vi "DataLog_Update.vi"() -> ()   [LabVIEW 2018]
panel:
  out "레코드":T1(array[cluster])
  in  "version 폴더 경로":path
  in  "정지 버튼":bool
  in  "업로드버튼":bool
  in  "업로드할 파일 정보 입력란":T2
  in  "데이터로그 경로(대화 상자 사용)":path
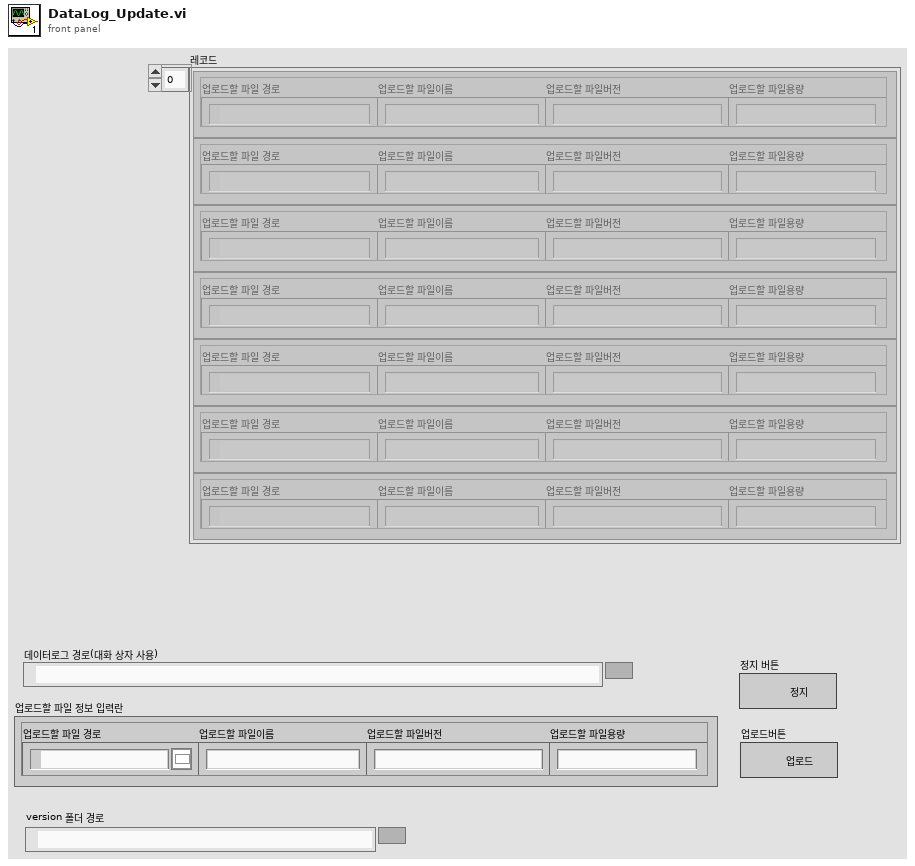
[diagram p1: front panel]
types:
  T1 = cluster{"업로드할 파일 경로":path, "업로드할 파일이름":string, "업로드할 파일버전":string, "업로드할 파일용량":string}[]
  T2 = cluster{"업로드할 파일 경로":path, "업로드할 파일이름":string, "업로드할 파일버전":string, "업로드할 파일용량":string}
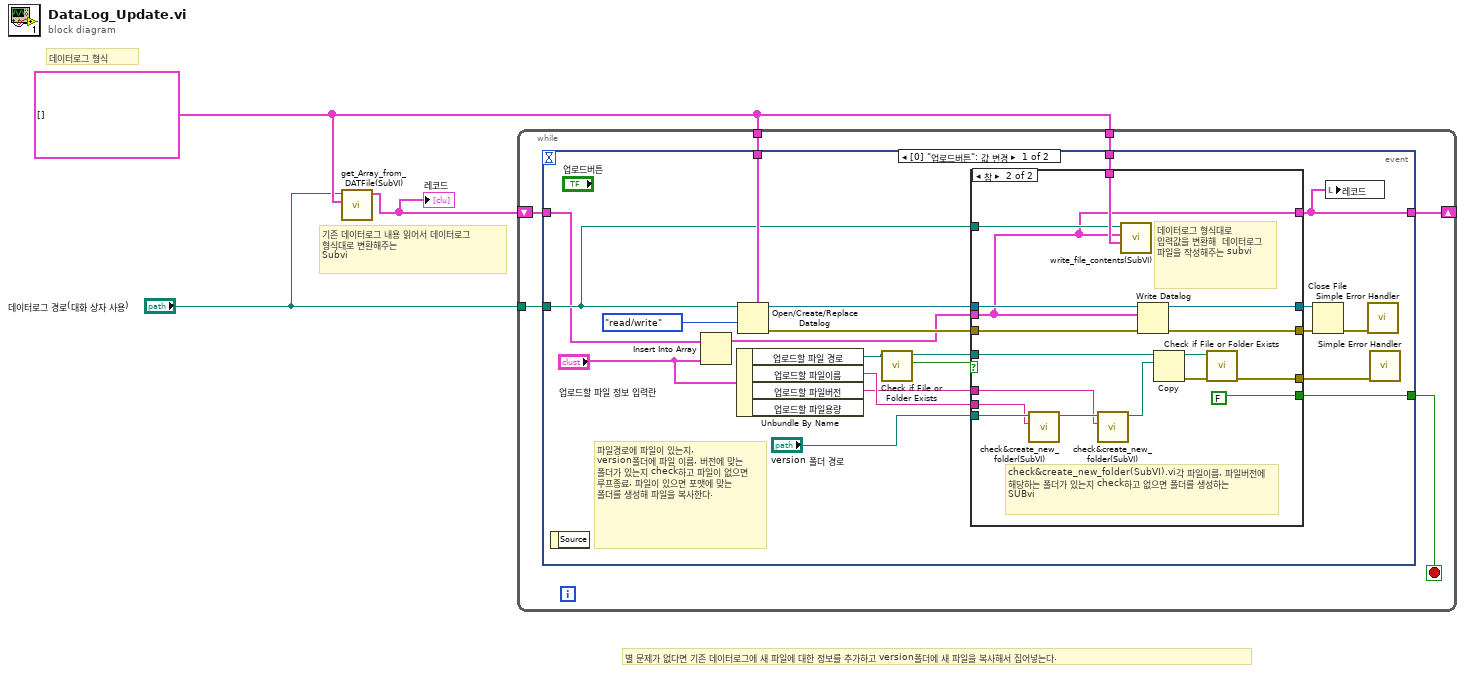
[diagram p0: block diagram]
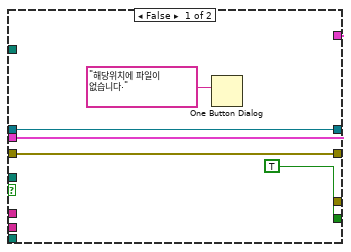
[diagram p2: hidden frame]
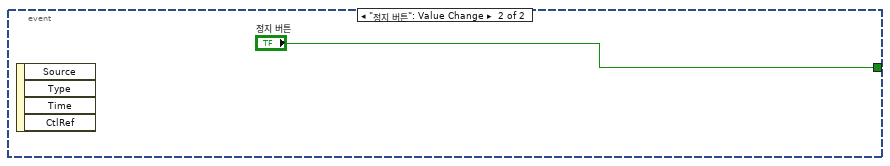
[diagram p3: hidden frame]
diagram:
  w3 = T1 [] ("레코드 2")
  # "데이터로그 형식"
  # "기존 데이터로그 내용 읽어서 데이터로그 형식대로 변환해주는\nSubvi"
  # "별 문제가 없다면 기존 데이터로그에 새 파일에 대한 정보를 추가하고 version폴더에 새 파일을 복사해서 집어넣는다."
  n1 = call "get_Array_from_DATFile(SubVI).vi"("레코드 3"=w3, "데이터로그 경로(대화 상자 사용)"="데이터로그 경로(대화 상자 사용)") -> ("레코드 2"=w1:T1)  [unwired: 9 in]
  "레코드" <- w1
  n2 = while {
    tunnel: w3 -> [w8]
    tunnel: "데이터로그 경로(대화 상자 사용)" -> [w7]
    tunnel: w3 -> [w6]
    shift-right: [w5] -> _
    shift-left: w1 -> [w4]
    stop <- w9 stop-if-true
    n3 = event shown="[0] \"업로드버튼\": 값 변경" {
      selector: _ -> [_ _]
      dyn-events: _ -> [_ _]
      timeout: _ -> [_ _]
      tunnel: [w19 "정지 버튼"] -> w9
      tunnel: w8 -> [w30 _]
      tunnel: w7 -> [w12 _]
      tunnel: w6 -> [w16 _]
      tunnel: w4 -> [w10 _]
      tunnel: [w11 _] -> w5
      event "업로드버튼": Value Change {
        # "파일경로에 파일이 있는지, \nversion폴더에 파일 이름, 버전에 맞는 폴더가 있는지 check하고 파일이 없으면 루프종료, 파일이 있으면 포맷에 맞는 폴더를 생성해 파일을 복사한다."
        n4 = event-data() -> ()  [unwired: 1 in, 1 out]
        n5 = Insert Into Array(array=w10, new element="업로드할 파일 정보 입력란") -> (w17:T1)  [unwired: 1 in]
        n6 = Unbundle By Name("업로드할 파일 정보 입력란") -> ("업로드할 파일 경로"=w13:path, "업로드할 파일이름"=w27:string, "업로드할 파일버전"=w26:string)  [unwired: 1 out]
        n7 = Open/Create/Replace Datalog(5:w30, 9:enum16{"read/write", "read-only", "write-only"}."read/write" ("접근(0:read/write)"), 11:w12) -> (0:w25:errorcluster, 3:w24:refnum<k1>)  [unwired: 3 in, 1 out]
        n8 = call <vilib>:"Check if File or Folder Exists.vi"("path"=w13) -> ("file or folder exists?"=w15:bool, "dup path"=w21:path)  [unwired: 8 in, 1 out]
        n9 = case shown="참" w15 {
          tunnel: [TRUE FALSE] -> w19
          tunnel: "version 폴더 경로" -> [_ w51]
          tunnel: w27 -> [_ w38]
          tunnel: w26 -> [_ w39]
          tunnel: w25 -> [w34 w49]
          tunnel: w17 -> [w31 w36]
          tunnel: w24 -> [w35 w48]
          tunnel: [w34 w47] -> w23
          tunnel: [w35 w46] -> w22
          tunnel: w21 -> [_ w44]
          tunnel: [_ w41] -> w20
          tunnel: w16 -> [_ w40]
          tunnel: w12 -> [_ w37]
          tunnel: [w31 w36] -> w11
          frame False {
            n10 = One Button Dialog(message="해당위치에 파일이 없습니다." ("메시지")) -> ()  [unwired: 1 in, 1 out]
          }
          frame True {
            # "데이터로그 형식대로 입력값을 변환해  데이터로그 파일을 작성해주는 subvi"
            # "check&create_new_folder(SubVI).vi각 파일이름, 파일버전에 해당하는 폴더가 있는지 check하고 없으면 폴더를 생성하는 SUBvi"
            n11 = call "check&create_new_folder(SubVI).vi"("업로드할 파일이름"=w38, "version 폴더 경로"=w51) -> ("dup path"=w50:path)  [unwired: 9 in]
            n12 = call "check&create_new_folder(SubVI).vi"("업로드할 파일이름"=w39, "version 폴더 경로"=w50) -> ("dup path"=w45:path)  [unwired: 9 in]
            n13 = call "write_file_contents(SubVI).vi"("레코드 3"=w40, "레코드 입력"=w36, "데이터로그 경로(대화 상자 사용)"=w37) -> ()  [unwired: 9 in]
            n14 = Write Datalog(4:w49, 6:w36, 7:w48) -> (0:w47:errorcluster, 3:w46:refnum<k1>)
            n15 = Copy(10:w45, 11:w44) -> (0:w42:errorcluster, 3:w43:path)  [unwired: 3 in, 1 out]
            n16 = call <vilib>:"Check if File or Folder Exists.vi"("error in (no error)"=w42, "path"=w43) -> ("error out"=w41:errorcluster)  [unwired: 7 in, 2 out]
          }
        }
        n17 = Close File(refnum=w22, error in=w23) -> (error out=w29:errorcluster)  [unwired: 1 out]
        n18 = local write "레코드"(w11) -> ()
        n19 = call <vilib>:"Simple Error Handler.vi"("error in (no error)"=w29) -> ()  [unwired: 4 in, 5 out]
        n20 = call <vilib>:"Simple Error Handler.vi"("error in (no error)"=w20) -> ()  [unwired: 4 in, 5 out]
      }
      event "정지 버튼": Value Change {
        n21 = event-data() -> ()  [unwired: 1 in, 4 out]
      }
    }
  }
